vi "gu_delete.vi"(8 "error in":errorcluster, 10 "Delete Hierarchy (F)":bool, 11 "Source Path":T1) -> (0 "error out":errorcluster)   [LabVIEW 2020, in "G-Unicode.lvlib"]
uses:
  G-Unicode.lvlib
  Types/Encoded UTF-8 String.ctl
  lib/g_unicode_32.dll
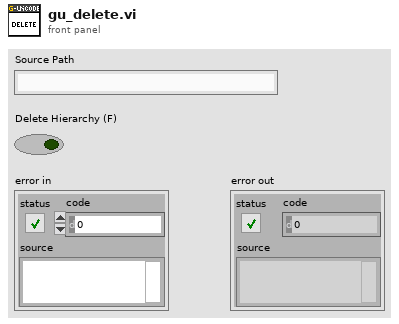
[diagram p1: front panel]
types:
  T1 = typedef "G-Unicode.lvlib/Encoded UTF-8 String.ctl" = string
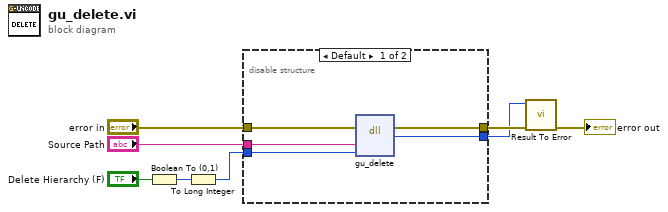
[diagram p0: block diagram]
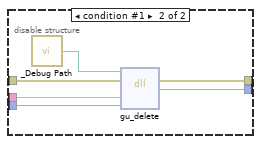
[diagram p2: hidden frame]
diagram:
  n1 = Boolean To (0,1)(Boolean="Delete Hierarchy (F)") -> (0, 1=w4:i16)
  n2 = To Long Integer(number=w4) -> (32bit integer=w3:i32)
  n3 = disable-structure shown="Default" {
    disable-tunnel: [w13 w19] -> w8
    disable-tunnel: [w12 w18] -> w1
    disable-tunnel: "Source Path" -> [w11 w17]
    disable-tunnel: "error in" -> [w10 w16]
    disable-tunnel: w3 -> [w9 w14]
    frame condition #0 (active) {
      n4 = dll-call lib="C:/github/dataflowg/g-unicode/src/LabVIEW/G-Unicode/lib/g_unicode_*.*" fn="gu_delete"(error in=w10, "source_path"=w11, "delete_hierarchy"=w9) -> (error out=w13:errorcluster, "result"=w12:i32)  [unwired: 4 in, 1 out]
    }
    frame condition #1 {
      n5 = call "_Debug Path.vi"() -> ("Debug Path"=w15:path)
      n6 = dll-call lib="?" fn="gu_delete"(path in=w15, error in=w16, "source_path"=w17, "delete_hierarchy"=w14) -> (error out=w19:errorcluster, "result"=w18:i32)  [unwired: 3 in, 1 out]
    }
  }
  n7 = call "Result To Error.vi"("error in (no error)"=w8, "Result Code"=w1) -> ("error out"=→"error out":errorcluster)  [unwired: 9 in]
